vi "Send Command Simplicity.vi"(5 "Message":string, 7 "Command":T1=enum."Start Run") -> (1 "Error":string, 3 "Data":string)   [LabVIEW 2015]
uses:
  Type/_Server Command.ctl
  Type/_Server Control Type.ctl
panel:
  out "Run Time (ms)":u32
  # "A DLL function to send a command to the Server"
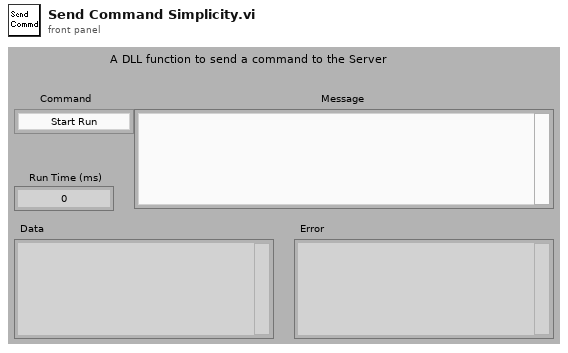
[diagram p1: front panel]
types:
  T1 = typedef "_Server Command.ctl" = enum16{"Hide Server", "Show Server", "Close Server", "Start Run", "Start Actual Run", "Stop Run", "Runtime Update", "Get Data", "Get Status", "Get Table", "Set Table", "Get Configuration", "Reserved", "Get Memory Map", "Read ADC", "Set Oscillator", "Reboot", "Backup Firmware", "Update Firmware", "Auxiliary Update", "System Status", "Start System", "Shutdown System", "Start LC Equilibration", "Get LC Status", "Get LC Configuration", "Get LC Method Contents", "Rinse Autosampler", "Pump OnOff", "Oven OnOff", "Get LC Error", "Clear LC Error", "Lock Server", "Get Current Method", "Get Real Time Data", "Connect LC", "Disconnect LC"}
  T2 = typedef "_Server Control Type.ctl" = enum16{"Command", "Boolean", "Text"}
  T3 = typedef "_Server Reference.ctl" = cluster{"Server Reference":refnum<vi>, "Command Ref":refnum<vi>, "Message Ref":refnum<vi>, "Ready Ref":refnum<vi>, "Locked Ref":refnum<vi>, "Data Ref":refnum<vi>, "Error Ref":refnum<vi>, "Busy Ref":refnum<vi>}
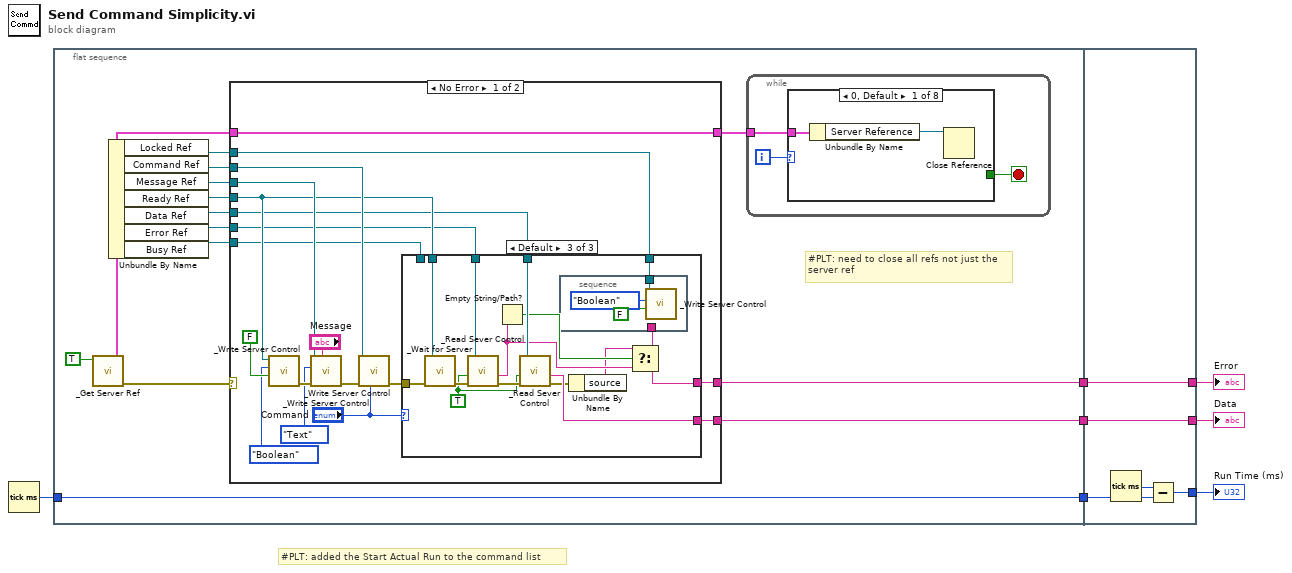
[diagram p0: block diagram]
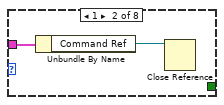
[diagram p2: hidden frame]
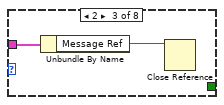
[diagram p3: hidden frame]
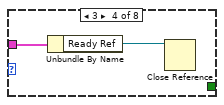
[diagram p4: hidden frame]
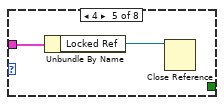
[diagram p5: hidden frame]
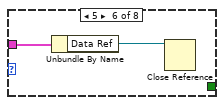
[diagram p6: hidden frame]
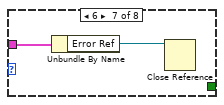
[diagram p7: hidden frame]
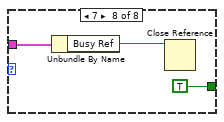
[diagram p8: hidden frame]
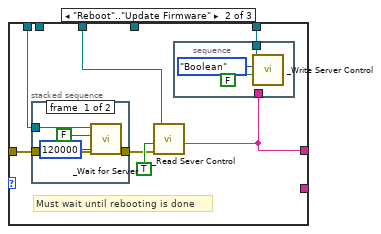
[diagram p10: hidden frame]
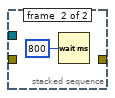
[diagram p11: hidden frame]
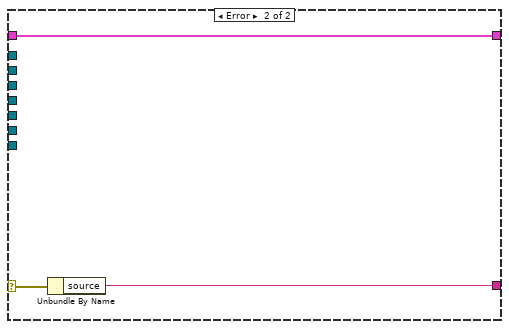
[diagram p12: hidden frame]
diagram:
  # "#PLT: added the Start Actual Run to the command list"
  n1 = Tick Count (ms)() -> (millisecond timer value=w7:u32)
  n2 = flat-sequence {
    tunnel: w7 -> [w12]
    tunnel: [w12] -> w6
    tunnel: [w9] -> w5
    tunnel: [w8] -> w4
    tunnel: w6 -> [w99]
    tunnel: w5 -> [w97]
    tunnel: w4 -> [w96]
    tunnel: [w98] -> w3
    tunnel: [w97] -> w2
    tunnel: [w96] -> w1
    frame #0 {
      # "#PLT: need to close all refs not just the\nserver ref"
      n3 = call "_Get Server Ref.vi"("IsSimplicityServer"=TRUE) -> ("error out"=w14:errorcluster, "Server Ref"=w11:T3)  [unwired: 5 out]
      n4 = Unbundle By Name(w11) -> ("Locked Ref"=w16:refnum<vi>, "Command Ref"=w17:refnum<vi>, "Message Ref"=w18:refnum<vi>, "Ready Ref"=w19:refnum<vi>, "Data Ref"=w20:refnum<vi>, "Error Ref"=w21:refnum<vi>, "Busy Ref"=w15:refnum<vi>)
      n5 = case shown="No Error" w14 {
        selector: w14 -> [_ w95]
        tunnel: [w44 w94] -> w9
        tunnel: [w55 _] -> w8
        tunnel: w17 -> [w53 _]
        tunnel: w18 -> [w54 _]
        tunnel: w19 -> [w52 _]
        tunnel: w20 -> [w48 _]
        tunnel: w21 -> [w49 _]
        tunnel: w16 -> [w43 _]
        tunnel: w15 -> [w45 _]
        tunnel: w11 -> [w42 w93]
        tunnel: [w42 w93] -> w10
        frame No Error {
          n6 = call "_Write Server Control.vi"("Boolean (F)"=FALSE, "Control Type"=_Server_Control_Type."Boolean", "Control Ref"=w52) -> ("error out"=w58:errorcluster)  [unwired: 4 in, 2 out]
          n7 = call "_Write Server Control.vi"("Text"="Message", "error in (no error)"=w58, "Control Type"=_Server_Control_Type."Text", "Control Ref"=w54) -> ("error out"=w57:errorcluster)  [unwired: 2 in, 3 out]
          n8 = call "_Write Server Control.vi"("Command"="Command", "error in (no error)"=w57, "Control Ref"=w53) -> ("error out"=w56:errorcluster)  [unwired: 3 in, 3 out]
          n9 = case shown="Default" "Command" {
            tunnel: w56 -> [_ w66 w89]
            tunnel: [_ _ w82] -> w55
            tunnel: w52 -> [_ _ w87]
            tunnel: w49 -> [_ w62 w86]
            tunnel: w48 -> [_ _ w83]
            tunnel: [_ w60 w76] -> w44
            tunnel: w45 -> [_ w65 _]
            tunnel: w43 -> [_ w61 w81]
            frame "Close Server" {
            }
            frame "Reboot".."Update Firmware" {
              # "Must wait until rebooting is done"
              n10 = stacked-sequence {
                tunnel: w66 -> [w74 _]
                tunnel: w65 -> [w73 _]
                tunnel: [w70 _] -> w63
                frame #0 {
                  n11 = call "_Wait for Server.vi"("error in"=w74, "Timeout (8s)"=u32 120000 ("Timeout (5s)"), "For Ready Signal? (T)"=FALSE, "Indicator Ref"=w73) -> ("error out"=w70:errorcluster)  [unwired: 3 out]
                }
                frame #1 {
                  n12 = Wait (ms)(milliseconds to wait=u32 800) -> ()  [unwired: 1 out]
                }
              }
              n13 = call "_Read Sever Control.vi"("error in (no error)"=w63, "Text? (F)"=TRUE, "Control Ref"=w62) -> ("Text"=w60:string)  [unwired: 1 in, 3 out]
              n14 = stacked-sequence {
                tunnel: w61 -> [w69]
                tunnel: w60 -> [_]
                frame #0 {
                  n15 = call "_Write Server Control.vi"("Boolean (F)"=FALSE, "Control Type"=_Server_Control_Type."Boolean", "Control Ref"=w69) -> ()  [unwired: 4 in, 3 out]
                }
              }
            }
            frame Default {
              w84 = TRUE
              n16 = call "_Wait for Server.vi"("error in"=w89, "Indicator Ref"=w87) -> ("error out"=w88:errorcluster)  [unwired: 2 in, 3 out]
              n17 = call "_Read Sever Control.vi"("error in (no error)"=w88, "Text? (F)"=w84, "Control Ref"=w86) -> ("error out"=w85:errorcluster, "Text"=w79:string)  [unwired: 1 in, 2 out]
              n18 = Empty String/Path?(string/path=w79) -> (empty?=w80:bool)
              n19 = call "_Read Sever Control.vi"("error in (no error)"=w85, "Text? (F)"=w84, "Control Ref"=w83) -> ("error out"=w78:errorcluster, "Text"=w82:string)  [unwired: 1 in, 2 out]
              n20 = Unbundle By Name(w78) -> ("source"=w77:string)
              n21 = Select(t=w77, s=w80, f=w79) -> (s? t:f=w76:string)
              n22 = stacked-sequence {
                tunnel: w81 -> [w92]
                tunnel: w76 -> [_]
                frame #0 {
                  n23 = call "_Write Server Control.vi"("Boolean (F)"=FALSE, "Control Type"=_Server_Control_Type."Boolean", "Control Ref"=w92) -> ()  [unwired: 4 in, 3 out]
                }
              }
            }
          }
        }
        frame Error {
          n24 = Unbundle By Name(w95) -> ("source"=w94:string)
        }
      }
      n25 = while {
        tunnel: w10 -> [w23]
        i -> [w24]
        stop <- w22 stop-if-true
        n26 = case shown="0, Default" w24 {
          tunnel: w23 -> [w26 w28 w30 w32 w34 w36 w38 w41]
          tunnel: [_ _ _ _ _ _ _ TRUE] -> w22
          frame 0, Default {
            n27 = Unbundle By Name(w26) -> ("Server Reference"=w25:refnum<vi>)
            n28 = Close Reference(reference=w25) -> ()  [unwired: 1 in, 1 out]
          }
          frame 1 {
            n29 = Unbundle By Name(w28) -> ("Command Ref"=w27:refnum<vi>)
            n30 = Close Reference(reference=w27) -> ()  [unwired: 1 in, 1 out]
          }
          frame 2 {
            n31 = Unbundle By Name(w30) -> ("Message Ref"=w29:refnum<vi>)
            n32 = Close Reference(reference=w29) -> ()  [unwired: 1 in, 1 out]
          }
          frame 3 {
            n33 = Unbundle By Name(w32) -> ("Ready Ref"=w31:refnum<vi>)
            n34 = Close Reference(reference=w31) -> ()  [unwired: 1 in, 1 out]
          }
          frame 4 {
            n35 = Unbundle By Name(w34) -> ("Locked Ref"=w33:refnum<vi>)
            n36 = Close Reference(reference=w33) -> ()  [unwired: 1 in, 1 out]
          }
          frame 5 {
            n37 = Unbundle By Name(w36) -> ("Data Ref"=w35:refnum<vi>)
            n38 = Close Reference(reference=w35) -> ()  [unwired: 1 in, 1 out]
          }
          frame 6 {
            n39 = Unbundle By Name(w38) -> ("Error Ref"=w37:refnum<vi>)
            n40 = Close Reference(reference=w37) -> ()  [unwired: 1 in, 1 out]
          }
          frame 7 {
            n41 = Unbundle By Name(w41) -> ("Busy Ref"=w40:refnum<vi>)
            n42 = Close Reference(reference=w40) -> ()  [unwired: 1 in, 1 out]
          }
        }
      }
    }
    frame #1 {
      n43 = Tick Count (ms)() -> (millisecond timer value=w100:u32)
      n44 = Subtract(x=w100, y=w99) -> (x-y=w98:u32)
    }
  }
  "Run Time (ms)" <- w3
  "Error" <- w2
  "Data" <- w1
